vi "SubVI de Flip Flop T (3).vi"(10 "Q1":bool, 11 "T":bool) -> (3 "Q1*":bool)   [LabVIEW 2018]
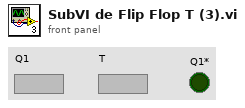
[diagram p1: front panel]
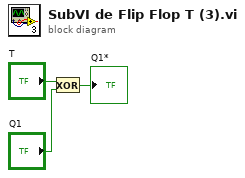
[diagram p0: block diagram]
diagram:
  n1 = Exclusive Or(1:"Q1", 2:"T") -> (0:→"Q1*":bool)
